vi "Find AI Channel Offsets and Update Settings.vi"(0 "DAQ":refnum<class "DAQ.lvclass">, 1 "AI channels update":string[](array[string])=["", "", "", "", "", "", ""], 5 "NumIterations (50)":i32=50, 7 "Test Progress ref":refnum<vi>, 9 "LoopInterval (100ms)":u32=100, 11 "error in (no error)":errorcluster) -> (4 "DAQ":refnum<class "DAQ.lvclass">, 15 "error out":errorcluster)   [LabVIEW 2017, in "DAQ.lvclass"]
doc: "Developed by Kevin Thompson\nkevin@thompsonengineering.net\n\nCopyright 2015\nThompson Engineering, LLC"
uses:
  DAQ.lvclass
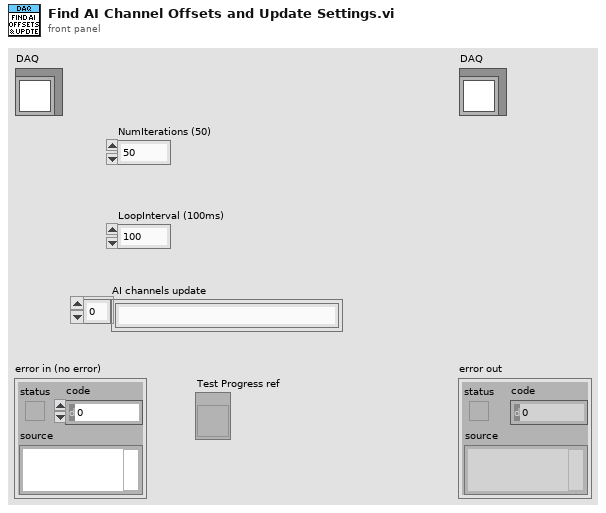
[diagram p1: front panel]
types:
  T1 = enum16{"Append", "Replace Last", "Flush All Previous"}
  T2 = cluster{"Status":enum16{"Working...", "Passed", "Failed", "Completed"}, "Action":enum16{"Start", "Check", "Valves", "Timer", "User Input", "Set", "End"}, "Mode":enum16{"Append", "Replace Last", "Flush All Previous"}}
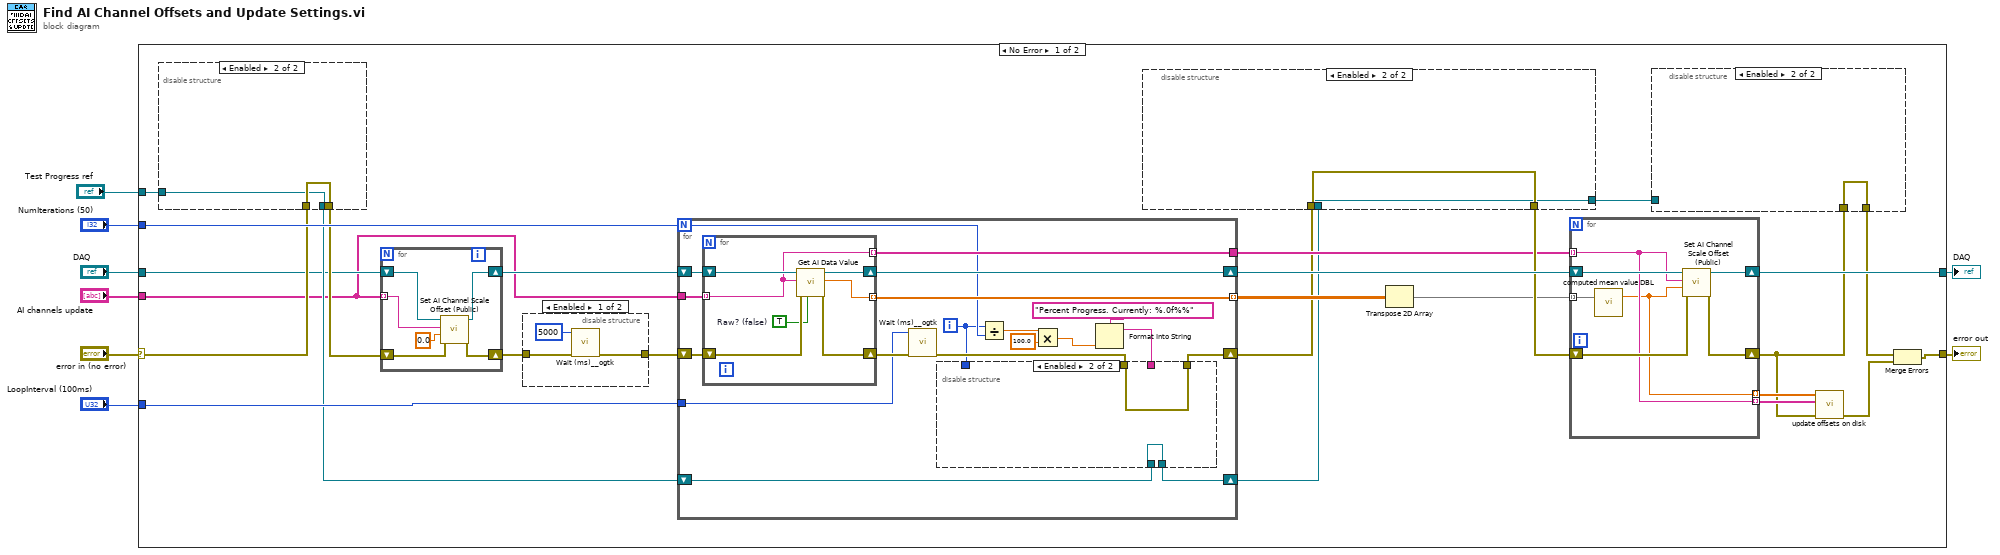
[diagram p0: block diagram]
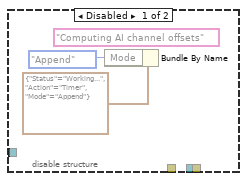
[diagram p2: hidden frame]
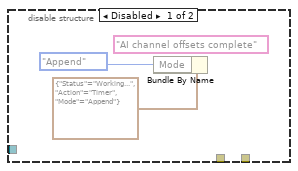
[diagram p3: hidden frame]
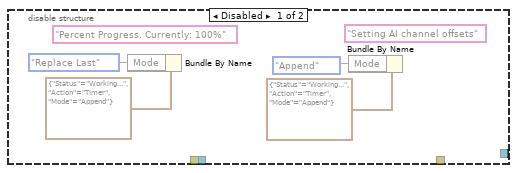
[diagram p4: hidden frame]
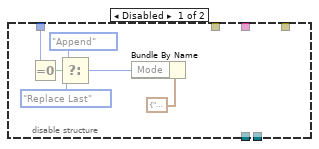
[diagram p6: hidden frame]
diagram:
  n1 = case shown="No Error" "error in (no error)" {
    selector: "error in (no error)" -> [w28 w119]
    tunnel: [w11 w119] -> w7
    tunnel: [w30 w118] -> w5
    tunnel: "DAQ" -> [w18 w118]
    tunnel: "NumIterations (50)" -> [w34 _]
    tunnel: "LoopInterval (100ms)" -> [w32 _]
    tunnel: "AI channels update" -> [w17 _]
    tunnel: "Test Progress ref" -> [w29 _]
    frame No Error {
      n2 = disable-structure shown="Enabled" {
        disable-tunnel: w29 -> [w39 w42]
        disable-tunnel: w28 -> [w38 w43]
        disable-tunnel: [w36 w42] -> w25
        disable-tunnel: [w35 w43] -> w20
        frame Disabled {
          w37 = "Computing AI channel offsets" ("Description (\"\")")
          n3 = Bundle By Name(cluster=T2 {"Status"=enum."Working...", "Action"=enum."Timer", "Mode"=enum."Append"} ("Progress settings cluster"), "Mode"=T1."Append") -> ()  [unwired: 1 out]
        }
        frame Enabled {
        }
      }
      n4 = for {
        tunnel: w17 -> [w67] mode=indexing
        shift-right: [w69] -> w16
        shift-left: w20 -> [w71]
        shift-right: [w70] -> w19
        shift-left: w18 -> [w72]
        n5 = call "Set AI Channel Scale Offset (Public).vi"("error in (no error)"=w71, "ScaleOffset"=0.0, "IOName"=w67, "DAQ"=w72) -> ("error out"=w69:errorcluster, "DAQ"=w70:refnum<class "DAQ.lvclass">)  [unwired: 6 in]
      }
      n6 = disable-structure shown="Enabled" {
        disable-tunnel: w16 -> [w65 w66]
        disable-tunnel: [w64 w66] -> w15
        frame Enabled {
          n7 = call <userlib>:"Wait (ms)__ogtk.vi"("error in (no error)"=w65, "milliseconds to wait"=u32 5000) -> ("error out"=w64:errorcluster)  [unwired: 8 in, 1 out]
        }
        frame Disabled {
        }
      }
      n8 = for {
        N: w34 -> [w74]
        shift-right: [w82] -> w21
        shift-left: w15 -> [w90]
        shift-right: [w89] -> w33
        shift-left: w19 -> [w91]
        tunnel: w32 -> [w87]
        tunnel: [w86] -> w31 mode=indexing
        tunnel: [w85] -> w26
        tunnel: w17 -> [w84]
        shift-right: [w81] -> w22
        shift-left: w25 -> [w80]
        i -> [w73]
        n9 = for {
          tunnel: [w107] -> w86 mode=indexing
          shift-right: [w108] -> w89
          shift-left: w91 -> [w110]
          shift-right: [w106] -> w88
          shift-left: w90 -> [w109]
          tunnel: [w105] -> w85 mode=indexing
          tunnel: w84 -> [w105] mode=indexing
          w104 = TRUE  # Raw? (false)
          n10 = call "Get AI Data Value.vi"("Raw? (false)"=w104, "error in (no error)"=w109, "AI IOName"=w105, "DAQ"=w110) -> ("error out"=w106:errorcluster, "Value"=w107:dbl, "DAQ"=w108:refnum<class "DAQ.lvclass">)  [unwired: 3 in, 2 out]
        }
        n11 = call <userlib>:"Wait (ms)__ogtk.vi"("error in (no error)"=w88, "milliseconds to wait"=w87) -> ("error out"=w83:errorcluster)  [unwired: 8 in, 1 out]
        n12 = Divide(x=w73, y=w74) -> (x/y=w77:dbl)
        n13 = Multiply(x=w77, y=100.0) -> (x*y=w75:dbl)
        n14 = Format Into String(format string="Percent Progress. Currently: %.0f%%" ("Description (\"\")"), w75) -> (resulting string=w78:string)  [unwired: 2 in, 1 out]
        n15 = disable-structure shown="Enabled" {
          disable-tunnel: w83 -> [w95 w103]
          disable-tunnel: [w94 w103] -> w82
          disable-tunnel: [_ w102] -> w81
          disable-tunnel: w80 -> [_ w102]
          disable-tunnel: w78 -> [w93 _]
          disable-tunnel: w73 -> [w92 _]
          frame Disabled {
            n16 = Equal To 0?(x=w92) -> (x = 0?=w99:bool)
            n17 = Select(t=T1."Append" ("Mode"), s=w99, f=T1."Replace Last" ("Mode")) -> (s? t:f=w96:T1)
            n18 = Bundle By Name(cluster=T2 {"Status"=enum."Working...", "Action"=enum."Timer", "Mode"=enum."Append"} ("Progress settings cluster"), "Mode"=w96) -> (w100:T2)
          }
          frame Enabled {
          }
        }
      }
      n19 = disable-structure shown="Enabled" {
        disable-tunnel: [w58 w62] -> w27
        disable-tunnel: [w57 w61] -> w24
        disable-tunnel: w22 -> [w54 w61]
        disable-tunnel: w21 -> [w53 w62]
        frame Disabled {
          w52 = "Percent Progress. Currently: 100%" ("Description (\"\")")
          w51 = "Setting AI channel offsets" ("Description (\"\")")
          n20 = Bundle By Name(cluster=T2 {"Status"=enum."Working...", "Action"=enum."Timer", "Mode"=enum."Append"} ("Progress settings cluster"), "Mode"=T1."Replace Last") -> ()  [unwired: 1 out]
          n21 = Bundle By Name(cluster=T2 {"Status"=enum."Working...", "Action"=enum."Timer", "Mode"=enum."Append"} ("Progress settings cluster"), "Mode"=T1."Append") -> ()  [unwired: 1 out]
        }
        frame Enabled {
        }
      }
      n22 = Transpose 2D Array(2D array=w31) -> (transposed array=w14:dbl[][])
      n23 = for {
        tunnel: w14 -> [w117] mode=indexing
        tunnel: w26 -> [w112] mode=indexing
        shift-right: [w113] -> w9
        shift-left: w27 -> [w115]
        shift-right: [w114] -> w30
        shift-left: w33 -> [w116]
        tunnel: [w112] -> w13 mode=indexing
        tunnel: [w111] -> w12 mode=indexing
        n24 = call <vilib>:"computed mean value DBL.vi"("Array in"=w117) -> ("MeanValue"=w111:dbl)  [unwired: 1 out]
        n25 = call "Set AI Channel Scale Offset (Public).vi"("error in (no error)"=w115, "ScaleOffset"=w111, "IOName"=w112, "DAQ"=w116) -> ("error out"=w113:errorcluster, "DAQ"=w114:refnum<class "DAQ.lvclass">)  [unwired: 6 in]
      }
      n26 = disable-structure shown="Enabled" {
        disable-tunnel: w24 -> [w46 _]
        disable-tunnel: [w45 w50] -> w23
        disable-tunnel: w9 -> [w44 w50]
        frame Disabled {
          w47 = "AI channel offsets complete" ("Description (\"\")")
          n27 = Bundle By Name(cluster=T2 {"Status"=enum."Working...", "Action"=enum."Timer", "Mode"=enum."Append"} ("Progress settings cluster"), "Mode"=T1."Append") -> ()  [unwired: 1 out]
        }
        frame Enabled {
        }
      }
      n28 = call "update offsets on disk.vi"("error in (no error)"=w9, "Offset IONames"=w13, "Offset Values"=w12) -> ("error out"=w10:errorcluster)  [unwired: 8 in]
      n29 = Merge Errors(w23, w10) -> (w11:errorcluster)
    }
    frame Error {
    }
  }
  "error out" <- w7
  "DAQ" <- w5
